vi "主动上传工控机周期和模式 (子VI).vi"() -> (3 "系统状态改变":bool)   [LabVIEW 2016, in "数据传输系统-05.lvlib"]
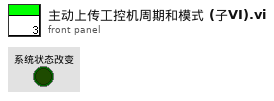
[diagram p1: front panel]
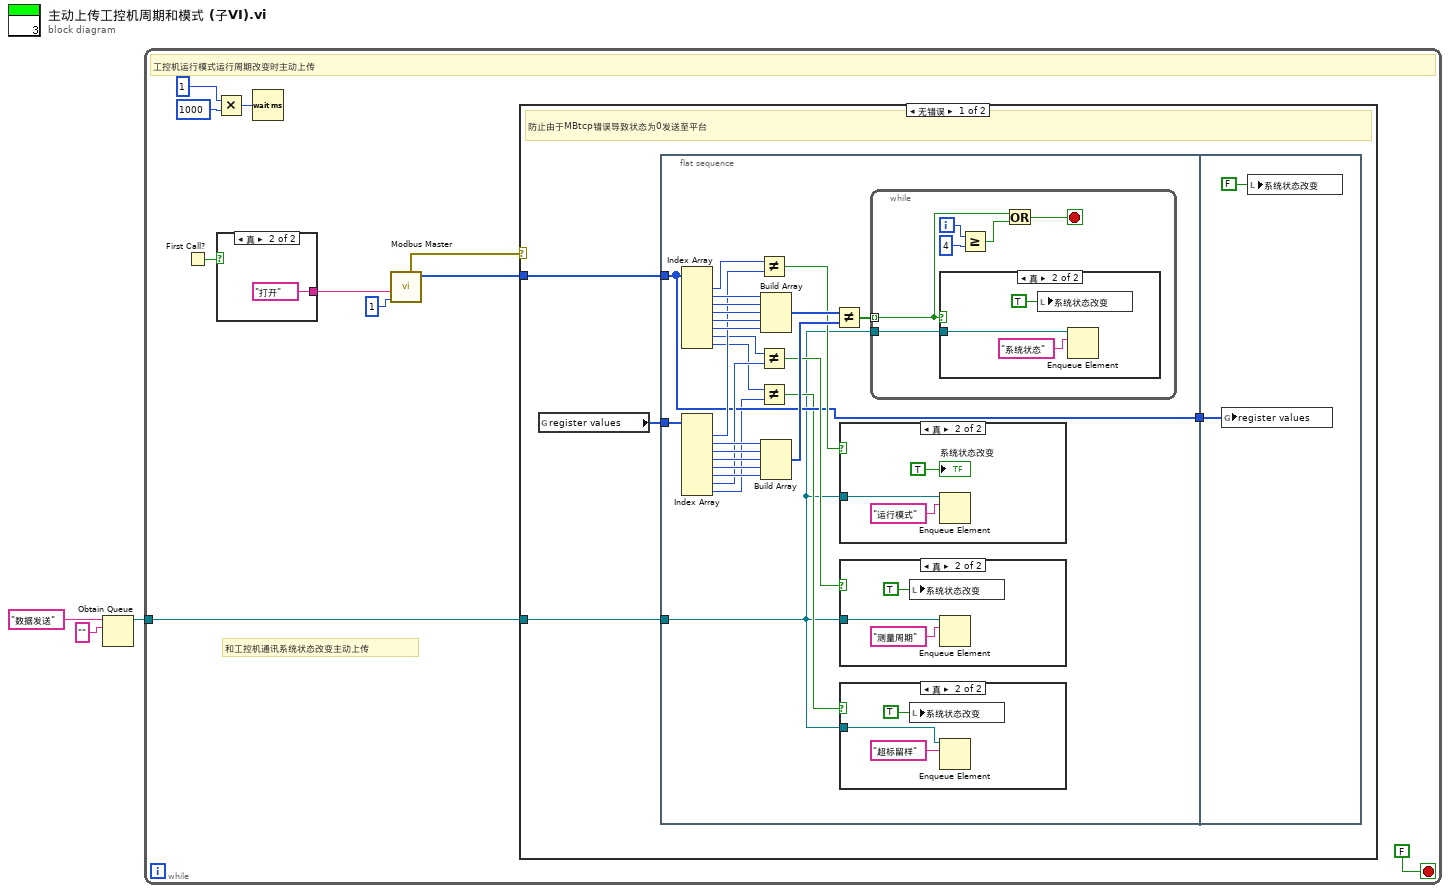
[diagram p0: block diagram]
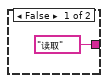
[diagram p7: hidden frame]
diagram:
  n1 = Obtain Queue(name (unnamed)="数据发送" ("名称（未命名）"), element data type="") -> (queue out=w3:refnum<queue>)  [unwired: 3 in, 2 out]
  n2 = while {
    tunnel: w3 -> [w6]
    stop <- FALSE stop-if-true
    # "和工控机通讯系统状态改变主动上传"
    # "工控机运行模式运行周期改变时主动上传"
    n3 = First Call?() -> (First Call?: T/F=w4:bool)
    n4 = Multiply(x=u32 1, y=u32 1000 ("等待时间（毫秒）")) -> (x*y=w12:u32)
    n5 = case shown="真" w4 {
      tunnel: ["读取" ("读取写入选择") "打开" ("读取写入选择")] -> w9
      frame False {
      }
      frame True {
      }
    }
    n6 = Wait (ms)(milliseconds to wait=w12) -> ()  [unwired: 1 out]
    n7 = call "Modbus Master.vi"("Unit ID"=u8 1, "读取写入选择"=w9) -> ("register values"=w7:u16[], "error out"=w5:errorcluster)  [unwired: 6 in, 2 out]
    n8 = case shown="无错误" w5 {
      tunnel: w7 -> [w16 _]
      tunnel: w6 -> [w14 _]
      frame No Error {
        # "防止由于MBtcp错误导致状态为0发送至平台"
        n9 = global read "全局1.vi" "register values"() -> (w15:u16[])
        n10 = flat-sequence {
          tunnel: w16 -> [w22]
          tunnel: w15 -> [w42]
          tunnel: w14 -> [w18]
          tunnel: [w22] -> w17
          tunnel: w17 -> [w62]
          frame #0 {
            n11 = Index Array(array=w22) -> (element #1=w29:u16, element #2=w41:u16, element #3=w40:u16, element #4=w39:u16, element #5=w38:u16, element #6=w37:u16, element #7=w27:u16, element #8=w21:u16)  [unwired: 8 in]
            n12 = Index Array(array=w42) -> (element #1=w28:u16, element #2=w36:u16, element #3=w35:u16, element #4=w34:u16, element #5=w33:u16, element #6=w32:u16, element #7=w26:u16, element #8=w20:u16)  [unwired: 8 in]
            n13 = Not Equal?(x=w29, y=w28) -> (x != y?=w24:bool)
            n14 = Not Equal?(x=w27, y=w26) -> (x != y?=w25:bool)
            n15 = Not Equal?(x=w21, y=w20) -> (x != y?=w19:bool)
            n16 = Build Array(w41, w40, w39, w38, w37) -> (w31:u16[])
            n17 = Build Array(w36, w35, w34, w33, w32) -> (w30:u16[])
            n18 = Not Equal?(x=w31, y=w30) -> (x != y?=w23:bool[])
            n19 = case shown="真" w24 {
              tunnel: w18 -> [_ w59]
              frame False {
              }
              frame True {
                n20 = Enqueue Element(queue=w59, element="运行模式" ("元素")) -> ()  [unwired: 2 in, 3 out]
                "系统状态改变" <- TRUE
              }
            }
            n21 = case shown="真" w25 {
              tunnel: w18 -> [_ w56]
              frame False {
              }
              frame True {
                n22 = local write "系统状态改变"(TRUE ("系统状态改变")) -> ()
                n23 = Enqueue Element(queue=w56, element="测量周期" ("元素")) -> ()  [unwired: 2 in, 3 out]
              }
            }
            n24 = case shown="真" w19 {
              tunnel: w18 -> [_ w44]
              frame False {
              }
              frame True {
                n25 = local write "系统状态改变"(TRUE ("系统状态改变")) -> ()
                n26 = Enqueue Element(queue=w44, element="超标留样" ("元素")) -> ()  [unwired: 2 in, 3 out]
              }
            }
            n27 = while {
              tunnel: w18 -> [w51]
              tunnel: w23 -> [w48] mode=indexing
              i -> [w50]
              stop <- w46 stop-if-true
              n28 = case shown="真" w48 {
                tunnel: w51 -> [_ w53]
                frame False {
                }
                frame True {
                  n29 = local write "系统状态改变"(TRUE ("系统状态改变")) -> ()
                  n30 = Enqueue Element(queue=w53, element="系统状态" ("元素")) -> ()  [unwired: 2 in, 3 out]
                }
              }
              n31 = Greater Or Equal?(x=w50, y=4) -> (x >= y?=w47:bool)
              n32 = Or(x=w48, y=w47) -> (x .or. y?=w46:bool)
            }
          }
          frame #1 {
            n33 = global write "全局1.vi" "register values"(w62) -> ()
            n34 = local write "系统状态改变"(FALSE ("系统状态改变")) -> ()
          }
        }
      }
      frame Error {
      }
    }
  }
